vi "Track Goal.vi"(7 "Original Image":T2(plugin-control), 9 "Camera Type":T3, 10 "Targets":T4(array[cluster]), 11 "Goal Display":T2(plugin-control)) -> (1 "Target Line Masking Out":T2(plugin-control), 2 "Best Target Available":T1, 3 "Found Targets":T5(array[cluster]) {"Normalized Rect"."Numeric 5" format="%#_2g"; "Normalized Rect"."Numeric 3" format="%#_2g"; "Normalized Rect"."Numeric 2" format="%#_2g"; "Normalized Rect"."Numeric" format="%#_2g"}, 5 "Goal Display":T2(plugin-control))   [LabVIEW 2015]
uses:
  Camera Types.ctl
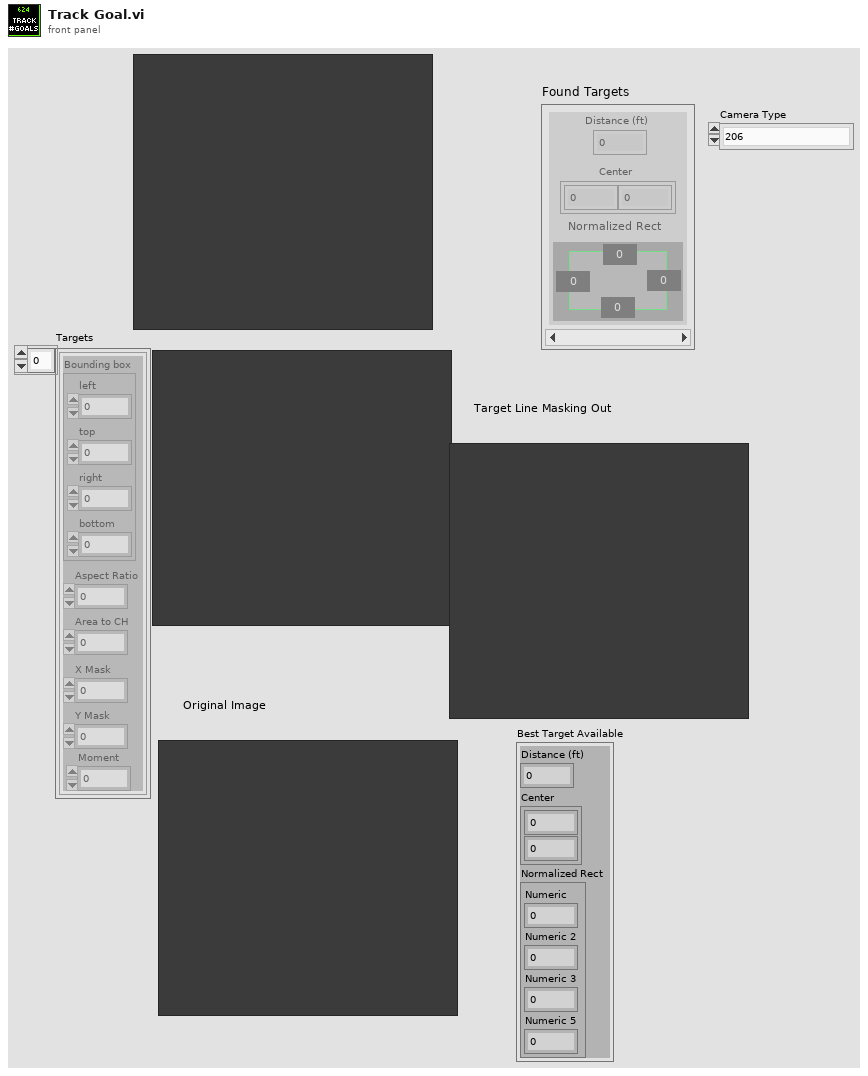
[diagram p1: front panel]
types:
  T1 = cluster{"Distance (ft)":dbl, "Center":cluster{dbl, dbl}, "Normalized Rect":cluster{"Numeric":dbl, "Numeric 2":dbl, "Numeric 3":dbl, "Numeric 5":dbl}}
  T2 = typedef "IMAQ Image.ctl" = refnum<image>
  T3 = typedef "Camera Types.ctl" = enum16{"206", "1011", "1013", "MS HD3000 square", "MS HD3000 640x480"}
  T4 = cluster{"Bounding box":cluster{"left":dbl, "top":dbl, "right":dbl, "bottom":dbl}, "Aspect Ratio":dbl, "Area to CH":dbl, "X Mask":dbl, "Y Mask":dbl, "Moment":dbl}[]
  T5 = cluster{"Distance (ft)":dbl, "Center":cluster{dbl, dbl}, "Normalized Rect":cluster{"Numeric":dbl, "Numeric 2":dbl, "Numeric 3":dbl, "Numeric 5":dbl}}[]
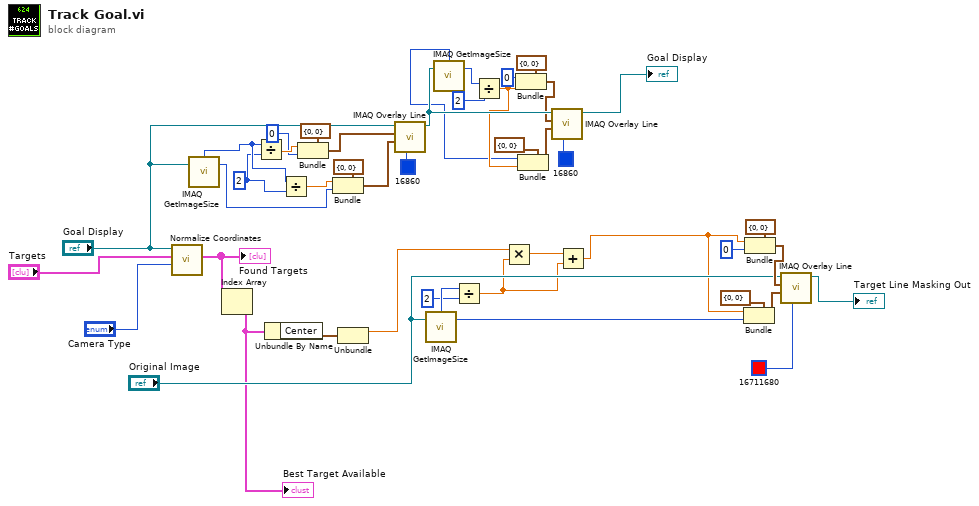
[diagram p0: block diagram]
diagram:
  w33 = 2 ("y")
  n1 = call "Normalize Coordinates.vi"("Camera Type"="Camera Type", "Targets"="Targets", "Image in"="Goal Display") -> ("Found Targets"=w10:T5)  [unwired: 7 in, 1 out]
  "Found Targets" <- w10
  n2 = call "IMAQ GetImageSize"("Image"="Goal Display") -> ("Y Resolution"=w31:i32, "X Resolution"=w34:i32)  [unwired: 3 in, 1 out]
  n3 = Index Array(array=w10) -> (element=w9:T1)  [unwired: 1 in]
  "Best Target Available" <- w9
  n4 = Divide(x=w34, y=w33) -> (x/y=w39:dbl)
  n5 = Unbundle By Name(w9) -> ("Center"=w8:cluster{dbl, dbl})
  n6 = Divide(x=w34, y=w33) -> (x/y=w37:dbl)
  n7 = Bundle(cluster=cluster{"X":i32, "Y":i32} {"X"=0, "Y"=0} ("Start Point"), "X"=w39, "Y"=0) -> (w35:cluster{"X":i32, "Y":i32})
  n8 = Bundle(cluster=cluster{"X":i32, "Y":i32} {"X"=0, "Y"=0} ("Start Point"), "X"=w37, "Y"=w31) -> (w32:cluster{"X":i32, "Y":i32})
  n9 = Unbundle(w8) -> (w4:dbl)  [unwired: 1 out]
  n10 = call "IMAQ Overlay Line"("Color"=u32 16860, "End Point"=w32, "Start Point"=w35, "Image"="Goal Display") -> ("Image Out"=w30:T2)  [unwired: 6 in, 1 out]
  n11 = call "IMAQ GetImageSize"("Image"="Original Image") -> ("Y Resolution"=w11:i32, "X Resolution"=w6:i32)  [unwired: 3 in, 1 out]
  n12 = call "IMAQ GetImageSize"("Image"=w30) -> ("Y Resolution"=w28:i32, "X Resolution"=w21:i32)  [unwired: 3 in, 1 out]
  n13 = Divide(x=w6, y=2) -> (x/y=w2:dbl)
  n14 = Divide(x=w28, y=2) -> (x/y=w22:dbl)
  n15 = Multiply(x=w4, y=w2) -> (x*y=w3:dbl)
  n16 = Bundle(cluster=cluster{"X":i32, "Y":i32} {"X"=0, "Y"=0} ("Start Point"), "X"=0, "Y"=w22) -> (w23:cluster{"X":i32, "Y":i32})
  n17 = Bundle(cluster=cluster{"X":i32, "Y":i32} {"X"=0, "Y"=0} ("Start Point"), "X"=w21, "Y"=w22) -> (w20:cluster{"X":i32, "Y":i32})
  n18 = call "IMAQ Overlay Line"("Color"=u32 16860, "End Point"=w20, "Start Point"=w23, "Image"=w30) -> ("Image Out"=→"Goal Display":T2)  [unwired: 6 in, 1 out]
  n19 = Add(x=w3, y=w2) -> (x+y=w1:dbl)
  n20 = Bundle(cluster=cluster{"X":i32, "Y":i32} {"X"=0, "Y"=0} ("Start Point"), "X"=w1, "Y"=w11) -> (w17:cluster{"X":i32, "Y":i32})
  n21 = Bundle(cluster=cluster{"X":i32, "Y":i32} {"X"=0, "Y"=0} ("Start Point"), "X"=w1, "Y"=0 ("X")) -> (w16:cluster{"X":i32, "Y":i32})
  n22 = call "IMAQ Overlay Line"("Color"=u32 16711680, "End Point"=w17, "Start Point"=w16, "Image"="Original Image") -> ("Image Out"=→"Target Line Masking Out":T2)  [unwired: 6 in, 1 out]
